vi "valve_init.vi"(7 "error in (no error)":errorcluster, 10 "VISA resource name":refnum<visa-resource-name>="COM1") -> (0 "error out":errorcluster, 1 "POSITIONS":string, 2 "ACTUATOR MODE":string, 3 "VISA resource name out":refnum<visa-resource-name>)   [LabVIEW 2013]
uses:
  <vilib>/Instr/_visa.llb/VISA Configure Serial Port (Instr).vi
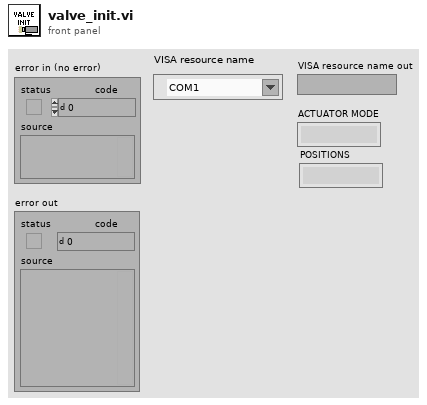
[diagram p1: front panel]
types:
  T1 = enum16{"Move to Home", "Set Positions", "Set Actuator Mode", "OTHER", "Set Direction", "CW Move", "CCW Move"}
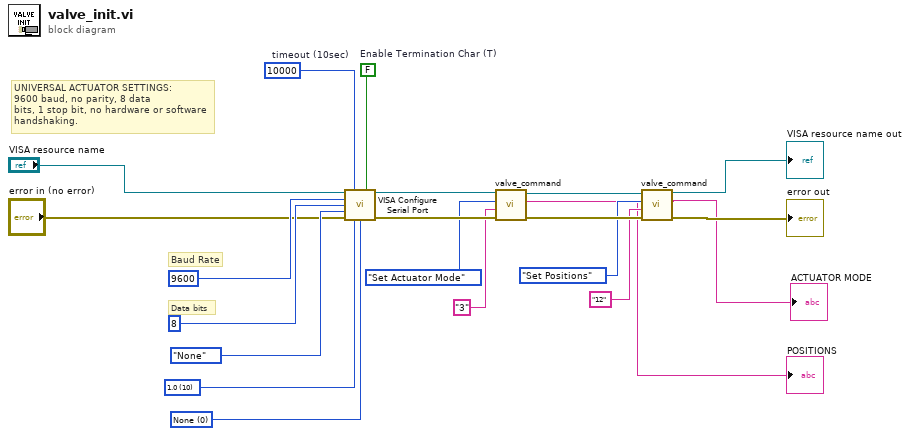
[diagram p0: block diagram]
diagram:
  w15 = u16 0 items=["None", "XON/XOFF", "RTS/CTS", "XON/XOFF & RTS/CTS", "DTR/DSR", "XON/XOFF & DTR/DSR"] ("flow control (0:none)")
  w16 = u16 10 items=["1.0"=10, "1.5"=15, "2.0"=20] ("stop bits (10: 1 bit)")
  w20 = FALSE  # Enable Termination Char (T)
  w21 = u32 10000  # timeout (10sec)
  # "UNIVERSAL ACTUATOR SETTINGS:\n9600 baud, no parity, 8 data \nbits, 1 stop bit, no hardware or software \nhandshaking."
  # "Data bits"
  # "Baud Rate"
  n1 = call-poly "VISA Configure Serial Port"("VISA resource name"="VISA resource name", "timeout (10sec)"=w21, "Enable Termination\nChar (T)"=w20, "baud rate (9600)"=u32 9600, "data bits (8)"=u16 8, "parity (0:none)"=enum16{"None", "Odd", "Even", "Mark", "Space"}."None", "error in (no error)"="error in (no error)", "stop bits (10: 1 bit)"=w16, "flow control (0:none)"=w15) -> ("VISA resource name out"=w14:refnum<visa-resource-name>, "error out"=w13:errorcluster)  [unwired: 5 in]
  n2 = call "valve_command.vi"("Error IN"=w13, "Command option"="3", "COMMANDS"=T1."Set Actuator Mode", "VALVE PORT IN"=w14) -> ("Error OUT"=w12:errorcluster, "read buffer"=→"POSITIONS":string, "VALVE PORT OUT"=w4:refnum<visa-resource-name>)  [unwired: 5 in]
  n3 = call "valve_command.vi"("Error IN"=w12, "Command option"="12", "COMMANDS"=T1."Set Positions", "VALVE PORT IN"=w4) -> ("Error OUT"=→"error out":errorcluster, "read buffer"=→"ACTUATOR MODE":string, "VALVE PORT OUT"=→"VISA resource name out":refnum<visa-resource-name>)  [unwired: 5 in]
